vi "sv_Swept Propagation Time.vi"(10 "board propagation time [samples]":dbl format="%#.1f", 11 "indice computations in":T1) -> (3 "indice computations in":T1)   [LabVIEW 2017, in "SoundVib_SweptSine.lvlib"]
uses:
  <vilib>/addons/Sound and Vibration/svt_Swept Sine/SoundVib_SweptSine.lvlib
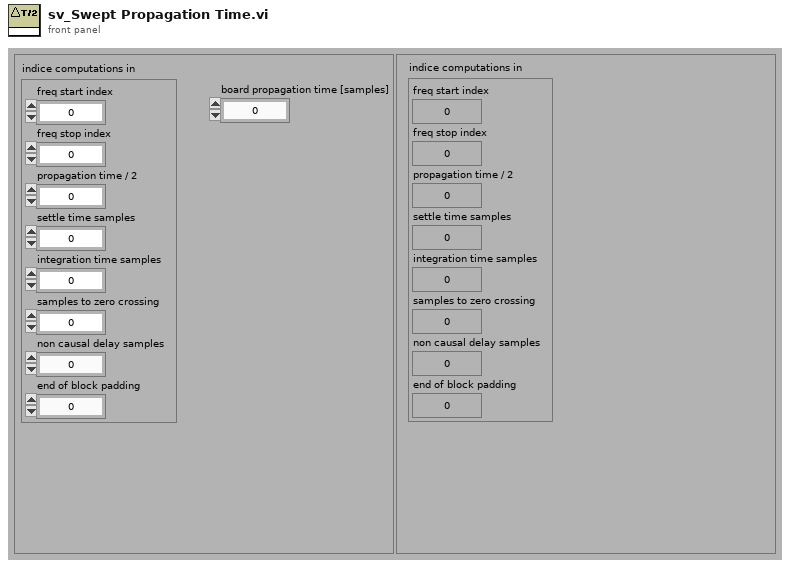
[diagram p1: front panel]
types:
  T1 = cluster{"freq start index":u32, "freq stop index":u32, "propagation time / 2":u32, "settle time samples":u32, "integration time samples":u32, "samples to zero crossing":u32, "non causal delay samples":u32, "end of block padding":u32}
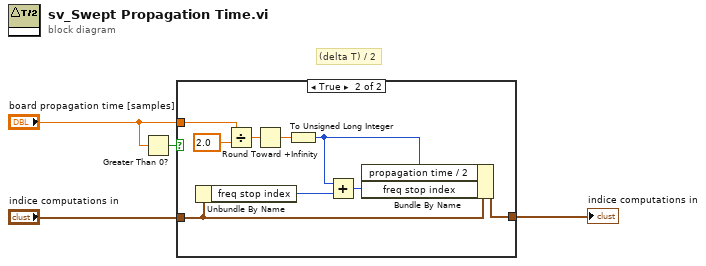
[diagram p0: block diagram]
diagram:
  # "(delta T) / 2"
  n1 = Greater Than 0?(x="board propagation time [samples]") -> (x > 0?=w4:bool)
  n2 = case shown="True" w4 {
    tunnel: "board propagation time [samples]" -> [_ w6]
    tunnel: "indice computations in" -> [w5 w10]
    tunnel: [w5 w7] -> w1
    frame False {
    }
    frame True {
      n3 = Unbundle By Name(w10) -> ("freq stop index"=w11:u32)
      n4 = Divide(x=w6, y=2.0) -> (x/y=w13:dbl)
      n5 = Round Toward +Infinity(x=w13) -> (ceil(x): smallest int >= x=w14:dbl)
      n6 = To Unsigned Long Integer(number=w14) -> (unsigned 32bit integer=w9:u32)
      n7 = Add(x=w9, y=w11) -> (x+y=w8:u32)
      n8 = Bundle By Name(cluster=w10, "propagation time / 2"=w9, "freq stop index"=w8) -> (w7:T1)
    }
  }
  "indice computations in" <- w1
